vi "Get All Names.vi"(9 "Active Plot":i32, 10 "Plot Name In":string[](array[string]), 11 "Multiplot Representation In":T2) -> (1 "Plot Range":T1, 2 "Plot Name Out":string[](array[string]), 3 "Multiplot Representation Out":T2)   [LabVIEW 2020, in "3D Plot.lvclass"]
uses:
  <vilib>/Math Plots/3D Math Plots/3D Plot/3D Plot/3D Plot.lvclass
  <vilib>/Math Plots/3D Math Plots/3D Plot/3D Plot/Typedef/Multiplot Representation.ctl
  <vilib>/Math Plots/3D Math Plots/3D Plot/3D Plot/Typedef/Plot Representation.ctl
  <vilib>/Math Plots/3D Math Plots/3D Plot/3D Plot/Typedef/Range Clusters.ctl
  <vilib>/Math Plots/3D Math Plots/3D Plot/3D Plot/Typedef/Mesh Data.ctl
panel:
  in  "Name Prefix":string="Plot "
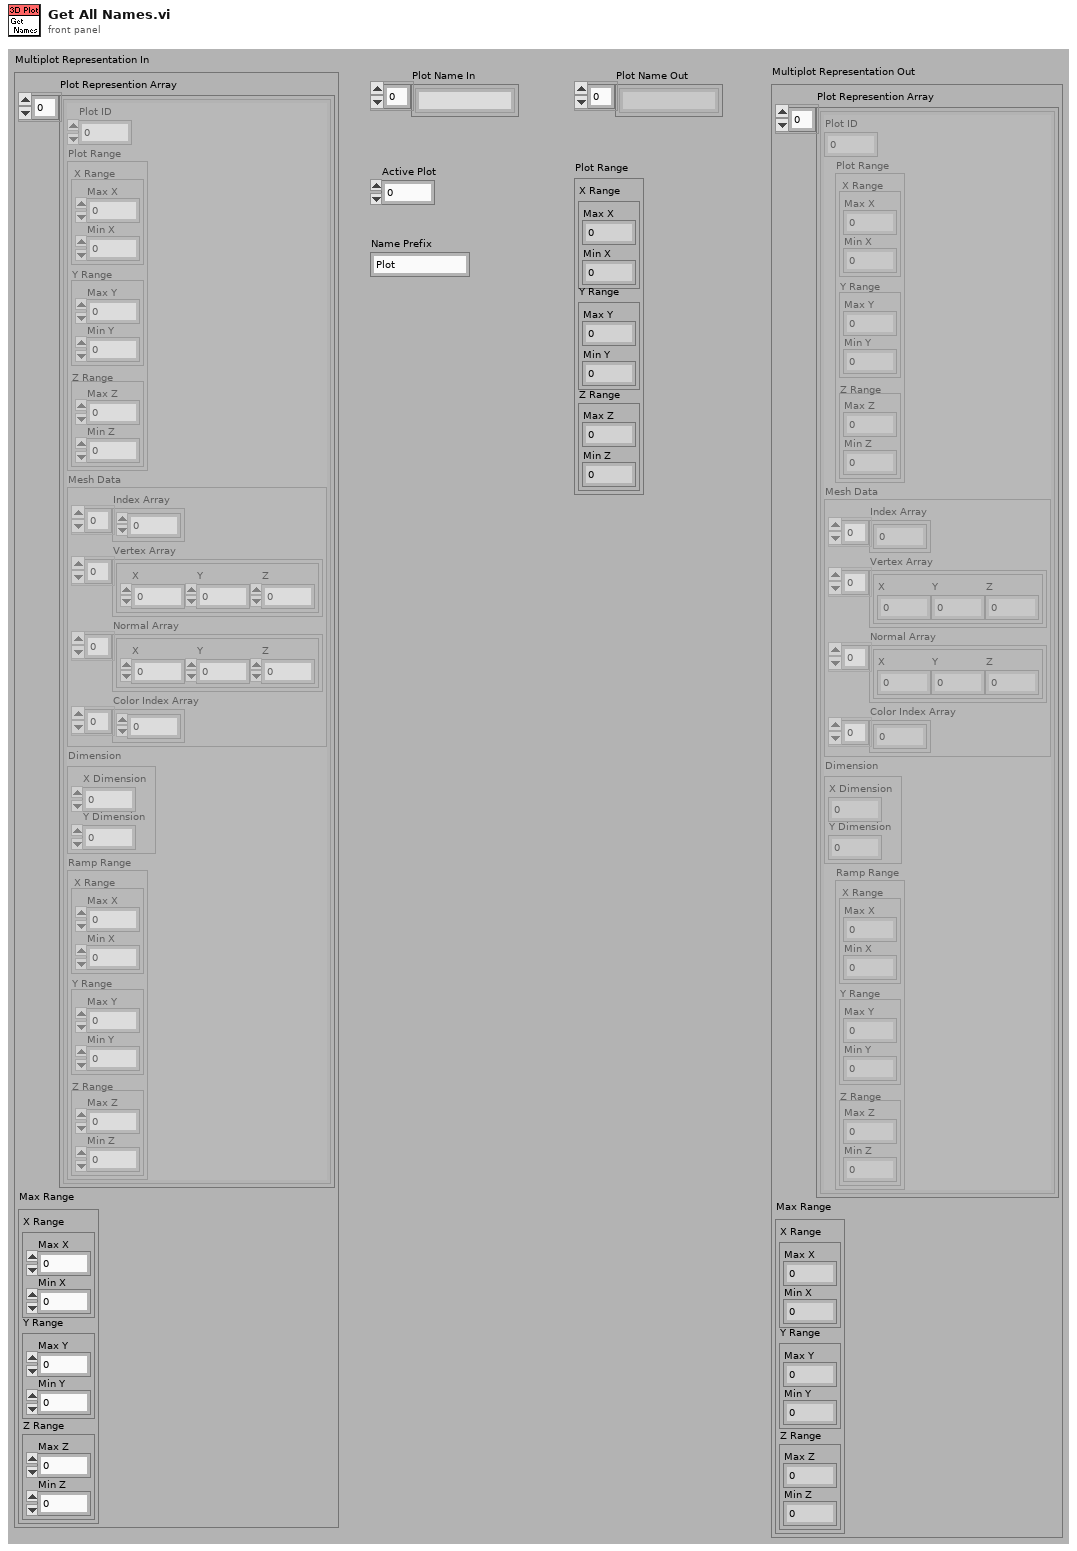
[diagram p1: front panel]
types:
  T1 = typedef "3D Plot.lvclass/Range Clusters.ctl" = cluster{"X Range":cluster{"Max X":sgl, "Min X":sgl}, "Y Range":cluster{"Max Y":sgl, "Min Y":sgl}, "Z Range":cluster{"Max Z":sgl, "Min Z":sgl}}
  T2 = typedef "3D Plot.lvclass/Multiplot Representation.ctl" = cluster{"Plot Represention Array":T3[], "Max Range":T1}
  T3 = typedef "3D Plot.lvclass/Plot Representation.ctl" = cluster{"Plot ID":i32, "Plot Range":T1, "Mesh Data":T4, "Dimension":cluster{"X Dimension":i32, "Y Dimension":i32}, "Ramp Range":T1}
  T4 = typedef "3D Plot.lvclass/Mesh Data.ctl" = cluster{"Index Array":u32[], "Vertex Array":cluster{"X":sgl, "Y":sgl, "Z":sgl}[], "Normal Array":cluster{"X":sgl, "Y":sgl, "Z":sgl}[], "Color Index Array":i32[]}
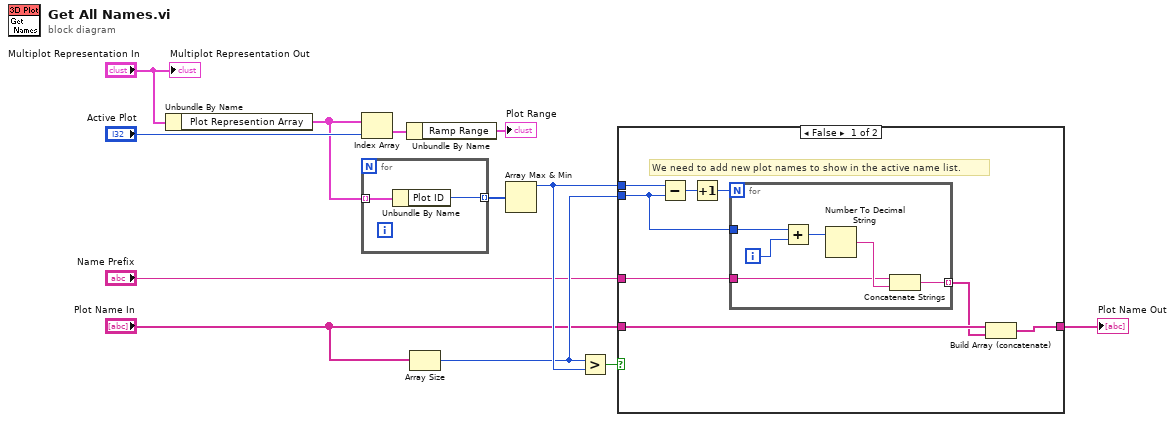
[diagram p0: block diagram]
diagram:
  n1 = Unbundle By Name("Multiplot Representation In") -> ("Plot Represention Array"=w11:T3[])
  n2 = Index Array(array=w11, index="Active Plot") -> (element=w10:T3)
  n3 = for {
    tunnel: w11 -> [w14] mode=indexing
    tunnel: [w13] -> w5 mode=indexing
    n4 = Unbundle By Name(w14) -> ("Plot ID"=w13:i32)
  }
  n5 = Unbundle By Name(w10) -> ("Ramp Range"=→"Plot Range":T1)
  n6 = Array Size(array="Plot Name In") -> (size(s)=w4:i32)
  n7 = Array Max & Min(array=w5) -> (max value=w7:i32)  [unwired: 3 out]
  n8 = Greater?(x=w4, y=w7) -> (0:w6:bool)
  n9 = case shown="False" w6 {
    tunnel: [w20 w29] -> w2
    tunnel: "Plot Name In" -> [w22 w29]
    tunnel: w4 -> [w16 _]
    tunnel: w7 -> [w17 _]
    tunnel: "Name Prefix" -> [w15 _]
    frame False {
      # "We need to add new plot names to show in the active name list."
      n10 = Subtract(x=w17, y=w16) -> (x-y=w19:i32)
      n11 = Increment(x=w19) -> (x+1=w18:i32)
      n12 = for {
        N: w18 -> [_]
        tunnel: w16 -> [w27]
        tunnel: [w24] -> w21 mode=indexing
        tunnel: w15 -> [w23]
        i -> [w28]
        n13 = Add(x=w27, y=w28) -> (x+y=w25:i32)
        n14 = Number To Decimal String(number=w25) -> (decimal integer string=w26:string)  [unwired: 1 out]
        n15 = Concatenate Strings(w23, w26) -> (w24:string)
      }
      n16 = Build Array (concatenate)(w22, w21) -> (w20:string[])
    }
    frame True {
      # "The plot with max ID can apply the stored name in the array."
    }
  }
  "Plot Name Out" <- w2
  "Multiplot Representation Out" <- "Multiplot Representation In"
